vi "Build.vi"(8 "error in (no error)":errorcluster, 11 "Class in":refnum<class "Installer.lvclass">) -> (0 "error out":errorcluster, 1 "GeneratedFiles out":path[](array[path]), 2 "GeneratedDirectories out":path[](array[path]), 3 "Class out":refnum<class "Installer.lvclass">)   [LabVIEW 2020, in "Installer.lvclass"]
uses:
  <vilib>/AppBuilder/IB_Classes/Installer/Installer.lvclass
  <vilib>/AppBuilder/IB_Classes/Installer/Installer.lvclass/Installer.ctl
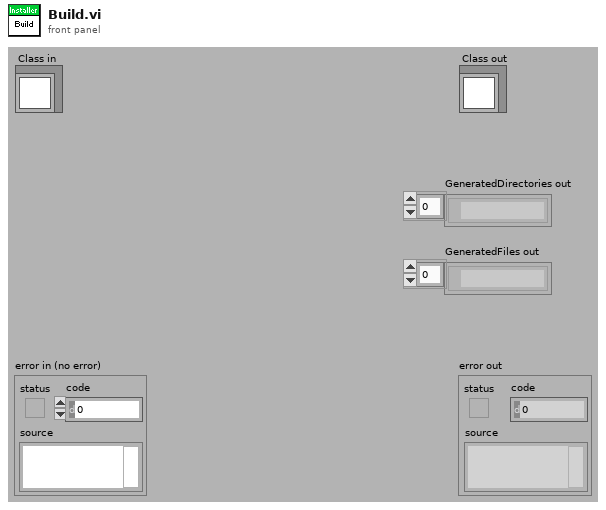
[diagram p1: front panel]
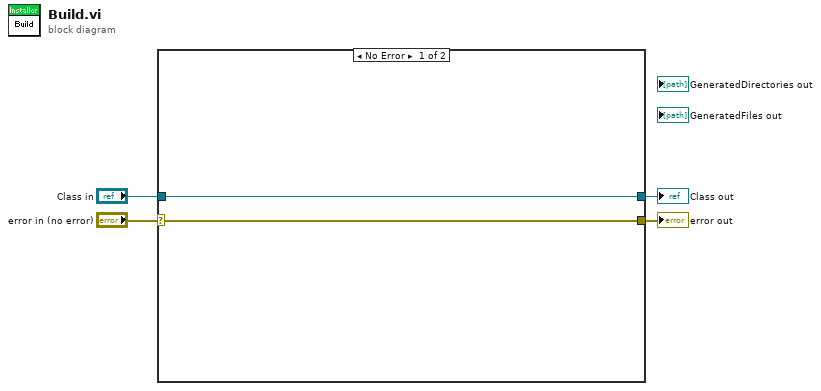
[diagram p0: block diagram]
diagram:
  n1 = case shown="No Error" "error in (no error)" {
    selector: "error in (no error)" -> [w5 w8]
    tunnel: [w5 w8] -> w1
    tunnel: [w6 w7] -> w2
    tunnel: "Class in" -> [w6 w7]
    frame No Error {
    }
    frame Error {
    }
  }
  "error out" <- w1
  "Class out" <- w2
